vi "decodeMap.vi"(8 "error in (no error)":errorcluster, 10 "ByteArray":u8[](array[numeric]) format="%.0x") -> (0 "error out":errorcluster, 2 "variant":variant, 3 "ByteArray":u8[](array[numeric]), 5 "Type":string)   [LabVIEW 2020, in "MsgPack.lvlib"]
uses:
  MsgPack.lvlib
  <vilib>/Utility/error.llb/Error Cluster From Error Code.vi
  <vilib>/ErrorRing/Error Ring.xnode
panel:
  out "Array":string[](array[string])
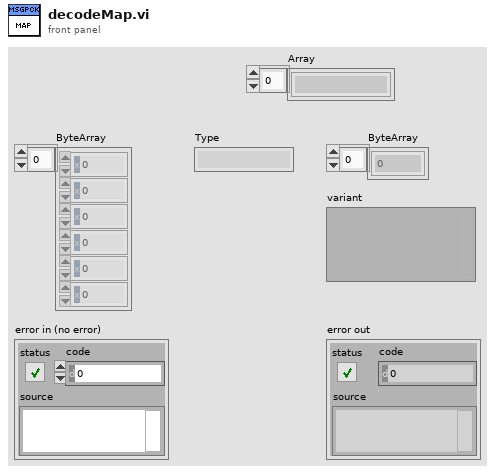
[diagram p1: front panel]
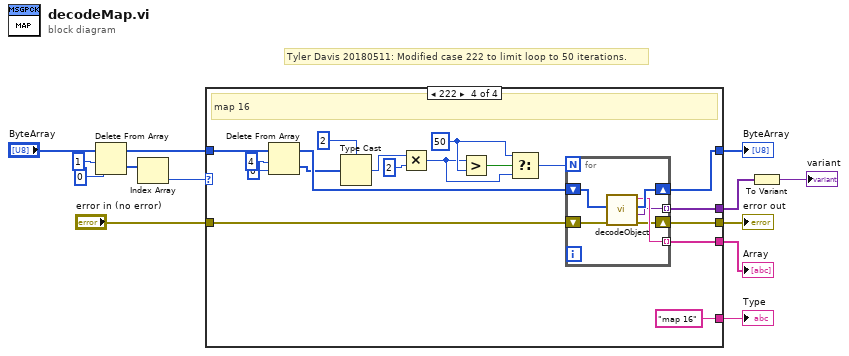
[diagram p0: block diagram]
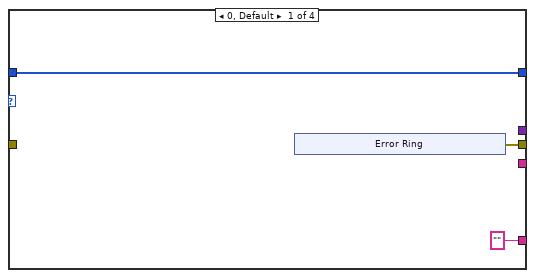
[diagram p2: hidden frame]
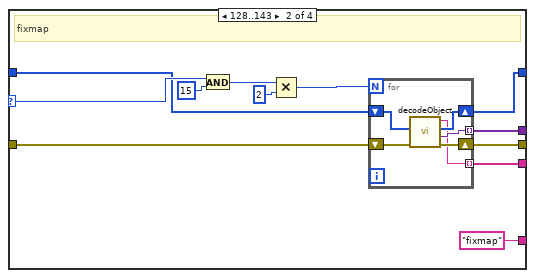
[diagram p3: hidden frame]
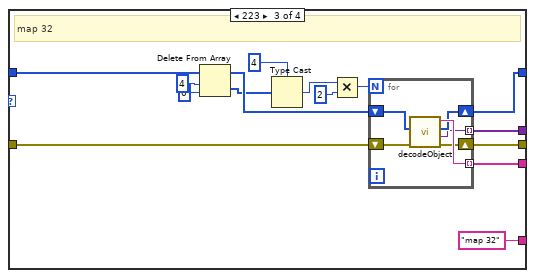
[diagram p4: hidden frame]
diagram:
  # "Tyler Davis 20180511: Modified case 222 to limit loop to 50 iterations."
  n1 = Delete From Array(array="ByteArray", length=1, index=0) -> (deleted portion=w4:u8[], array with subset deleted=w3:u8[])
  n2 = Index Array(array=w4) -> (element=w10:u8)  [unwired: 1 in]
  n3 = case shown="222" w10 {
    selector: w10 -> [_ w32 _ _]
    tunnel: [w16 w28 w52 w76] -> w12
    tunnel: "error in (no error)" -> [_ w29 w53 w77]
    tunnel: ["" "fixmap" "map 32" "map 16"] -> w9
    tunnel: [_ w27 w51 w75] -> w8
    tunnel: w3 -> [w14 w30 w49 w73]
    tunnel: [_ w26 w50 w74] -> w7
    tunnel: [w14 w25 w44 w68] -> w2
    frame 0, Default {
      n4 = xnode "Error Ring"() -> ("error out"=w16:errorcluster)
    }
    frame 128..143 {
      # "fixmap"
      n5 = And(x=w32, y=u8 15) -> (x .and. y?=w23:u8)
      n6 = Multiply(x=w23, y=u8 2) -> (x*y=w22:u8)
      n7 = for {
        N: w22 -> [_]
        shift-right: [w36] -> w25
        shift-left: w30 -> [w34]
        tunnel: [w35] -> w26 mode=indexing
        shift-right: [w38] -> w28
        shift-left: w29 -> [w39]
        tunnel: [w37] -> w27 mode=indexing
        n8 = call "decodeObject.vi"("error in (no error)"=w39, "ByteArray"=w34) -> ("error out"=w38:errorcluster, "Variant"=w37:variant, "RemainingBytes"=w36:u8[], "Type"=w35:string)  [unwired: 6 in]
      }
    }
    frame 223 {
      # "map 32"
      n9 = Delete From Array(array=w49, length=4, index=0) -> (deleted portion=w46:u8[], array with subset deleted=w47:u8[])
      n10 = Type Cast(type=u32 4 ("length"), x=w46) -> (*(type *) &x=w42:u32)
      n11 = Multiply(x=w42, y=u8 2) -> (x*y=w41:u32)
      n12 = for {
        N: w41 -> [_]
        shift-right: [w57] -> w44
        shift-left: w47 -> [w59]
        tunnel: [w58] -> w50 mode=indexing
        shift-right: [w55] -> w52
        shift-left: w53 -> [w60]
        tunnel: [w56] -> w51 mode=indexing
        n13 = call "decodeObject.vi"("error in (no error)"=w60, "ByteArray"=w59) -> ("error out"=w55:errorcluster, "Variant"=w56:variant, "RemainingBytes"=w57:u8[], "Type"=w58:string)  [unwired: 6 in]
      }
    }
    frame 222 {
      w63 = u32 50 ("y")
      # "map 16"
      n14 = Delete From Array(array=w73, length=4, index=0) -> (deleted portion=w70:u8[], array with subset deleted=w71:u8[])
      n15 = Type Cast(type=u32 2 ("length"), x=w70) -> (*(type *) &x=w66:u32)
      n16 = Multiply(x=w66, y=u8 2) -> (x*y=w62:u32)
      n17 = Greater?(x=w62, y=w63) -> (0:w64:bool)
      n18 = Select(t=w63, s=w64, f=w62) -> (s? t:f=w61:u32)
      n19 = for {
        N: w61 -> [_]
        shift-right: [w83] -> w68
        shift-left: w71 -> [w84]
        tunnel: [w82] -> w74 mode=indexing
        shift-right: [w80] -> w76
        shift-left: w77 -> [w79]
        tunnel: [w81] -> w75 mode=indexing
        n20 = call "decodeObject.vi"("error in (no error)"=w79, "ByteArray"=w84) -> ("error out"=w80:errorcluster, "Variant"=w81:variant, "RemainingBytes"=w83:u8[], "Type"=w82:string)  [unwired: 6 in]
      }
    }
  }
  "error out" <- w12
  "Type" <- w9
  "Array" <- w7
  "ByteArray" <- w2
  n21 = To Variant(anything=w8) -> (Variant=→"variant":variant)
